vi "Generate Getter VI.vi"(8 "error in (no error)":errorcluster, 9 "class path":path, 10 "Attribute Name":string) -> (0 "error out":errorcluster)   [LabVIEW 2020, in "Method Generation.lvlib" / "Getter Generator.lvclass"]
uses:
  Getter Generator.lvclass
  Getter Generator.lvclass/Getter Generator.ctl
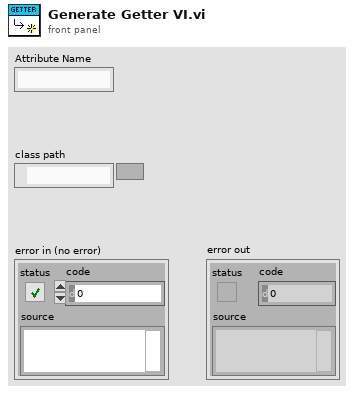
[diagram p1: front panel]
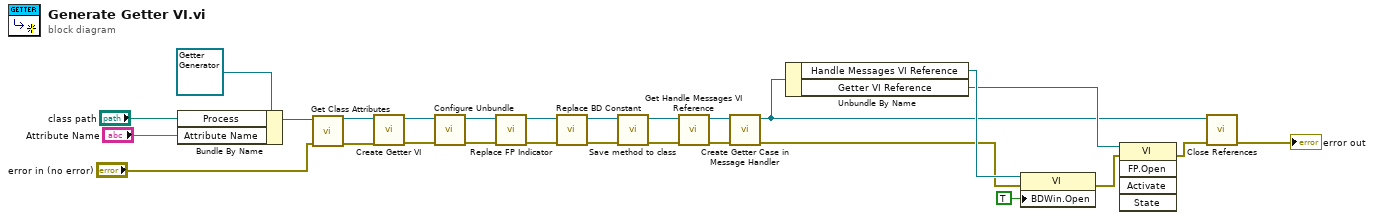
[diagram p0: block diagram]
diagram:
  n1 = Bundle By Name(cluster=refnum<class "Getter Generator.lvclass"> refnum ("New Getter Dialog In"), "Process"="class path", "Attribute Name"="Attribute Name") -> (w18:refnum<class "Getter Generator.lvclass">)
  n2 = call "Get Class Attributes.vi"("error in (no error)"="error in (no error)", "New Getter Dialog In"=w18) -> ("error out"=w23:errorcluster, "New Getter Dialog Out"=w21:refnum<class "Getter Generator.lvclass">)  [unwired: 8 in]
  n3 = call "Create Getter VI.vi"("error in (no error)"=w23, "New Getter Dialog in"=w21) -> ("error out"=w25:errorcluster, "New Getter Dialog out"=w22:refnum<class "Getter Generator.lvclass">)  [unwired: 8 in]
  n4 = call "Configure Unbundle.vi"("error in (no error)"=w25, "Getter Generator in"=w22) -> ("error out"=w16:errorcluster, "Getter Generator out"=w26:refnum<class "Getter Generator.lvclass">)  [unwired: 8 in]
  n5 = call "Replace FP Indicator.vi"("error in (no error)"=w16, "Getter Generator In"=w26) -> ("error out"=w15:errorcluster, "Getter Generator Out"=w27:refnum<class "Getter Generator.lvclass">)  [unwired: 8 in]
  n6 = call "Replace BD Constant.vi"("error in (no error)"=w15, "Getter Generator In"=w27) -> ("error out"=w13:errorcluster, "Getter Generator Out"=w12:refnum<class "Getter Generator.lvclass">)  [unwired: 8 in]
  n7 = call "Save method to class.vi"("error in (no error)"=w13, "Getter Generator In"=w12) -> ("error out"=w9:errorcluster, "Getter Generator Out"=w10:refnum<class "Getter Generator.lvclass">)  [unwired: 8 in]
  n8 = call "Get Handle Messages VI Reference.vi"("error in (no error)"=w9, "Getter Generator in"=w10) -> ("error out"=w11:errorcluster, "Getter Generator out"=w8:refnum<class "Getter Generator.lvclass">)  [unwired: 8 in]
  n9 = call "Create Getter Case in Message Handler.vi"("error in (no error)"=w11, "Getter Generator in"=w8) -> ("error out"=w3:errorcluster, "Getter Generator out"=w4:refnum<class "Getter Generator.lvclass">)  [unwired: 8 in]
  n10 = Unbundle By Name(w4) -> ("Handle Messages VI Reference"=w7:refnum<vi>, "Getter VI Reference"=w5:refnum<vi>)
  n11 = property class="VI"(reference=w7, error in=w3, "BDWin.Open"=TRUE ("Block Diagram Window:Open")) -> (error out=w2:errorcluster)  [unwired: 1 out]
  n12 = invoke class="VI" method="FP.Open"(reference=w5, error in=w2) -> (error out=w1:errorcluster)  [unwired: 3 in, 4 out]
  n13 = call "Close References.vi"("error in (no error)"=w1, "Getter Generator in"=w4) -> ("error out"=→"error out":errorcluster)  [unwired: 9 in]
